vi "Upload to Sift.vi"(0 "API GRPC URL":string, 1 "Absolute Filepath":path, 5 "API Key":string, 7 "error in (no error)":errorcluster, 9 "Asset Name":string="LabVIEW-TDMS-Example", 11 "Run Name":string="TDMS Upload Example", 12 "API REST URL":string) -> (4 "Run URL":string, 15 "Error":errorcluster)   [LabVIEW 2024, in "Sift TDMS Uploader.lvlib" / "Sift TDMS Uploader.lvclass"]
doc: "Uploads TDMS file to Sift with provided Run and Asset"
uses:
  Sift TDMS Uploader.lvclass
  <vilib>/Sift/Sift/Sift API/Sift Client.lvclass
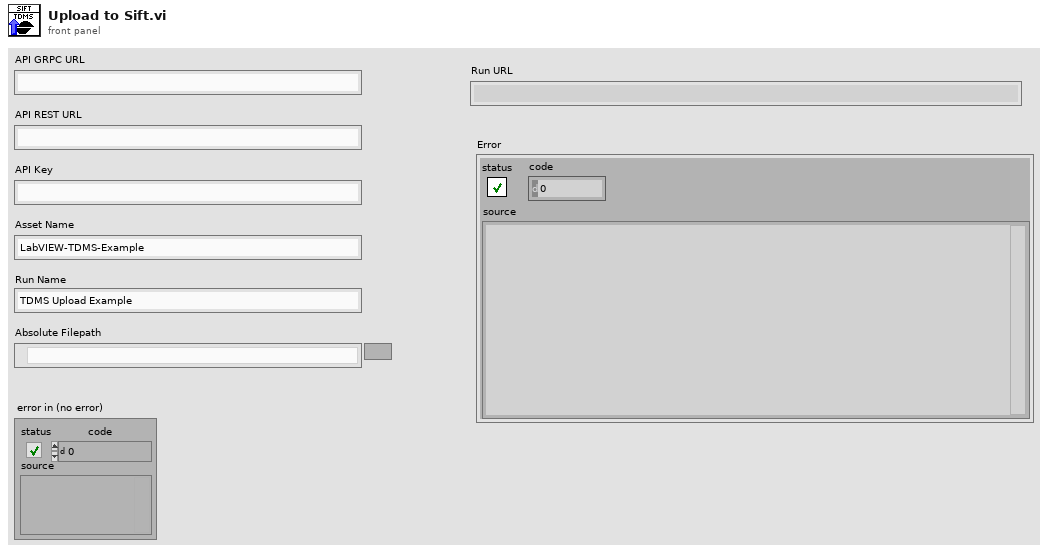
[diagram p1: front panel]
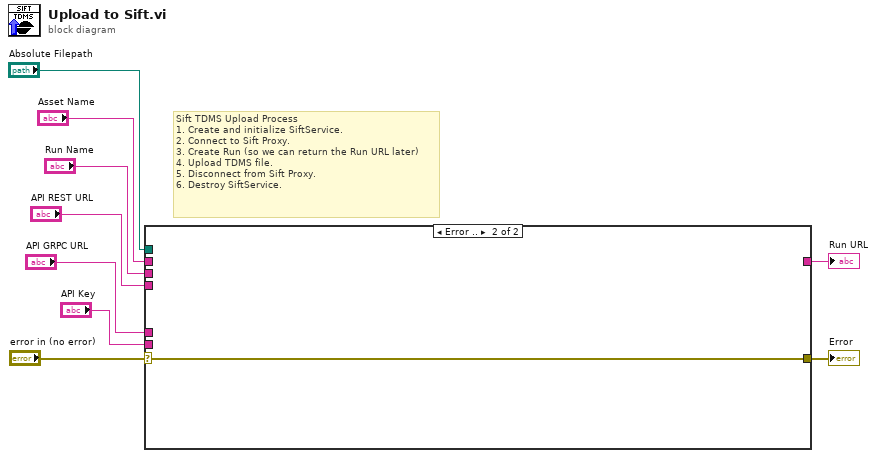
[diagram p0: block diagram]
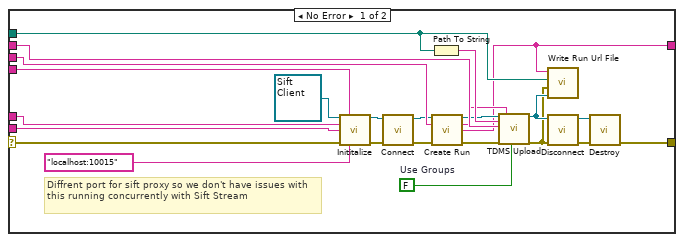
[diagram p2: hidden frame]
diagram:
  # "Sift TDMS Upload Process\n1. Create and initialize SiftService.\n2. Connect to Sift Proxy.\n3. Create Run (so we can return the Run URL later)\n4. Upload TDMS file.\n5. Disconnect from Sift Proxy.\n6. Destroy SiftService."
  n1 = case shown="Error .." "error in (no error)" {
    selector: "error in (no error)" -> [w12 w34]
    tunnel: [w32 w34] -> w9
    tunnel: "Asset Name" -> [w28 _]
    tunnel: "API GRPC URL" -> [w25 _]
    tunnel: "API Key" -> [w24 _]
    tunnel: "API REST URL" -> [w23 _]
    tunnel: "Run Name" -> [w22 _]
    tunnel: "Absolute Filepath" -> [w16 _]
    tunnel: [w15 _] -> w2
    frame No Error {
      w10 = FALSE  # Use Groups
      # "Diffrent port for sift proxy so we don't have issues with this running concurrently with Sift Stream"
      n2 = call-dynamic "Inititalize.vi"("Sift Client in"=refnum<class "Sift Client.lvclass"> refnum ("Sift Client.lvlib:Sift Client.lvclass"), "REST URL"=w23, "GRPC URL"=w25, "API Key"=w24, "error in (no error)"=w12, "Sift Proxy Address"="localhost:10015") -> ("Sift Client out"=w31:refnum<class "Sift Client.lvclass">, "error out"=w26:errorcluster)  [unwired: 8 in]
      n3 = call-dynamic "Connect.vi"("error in (no error)"=w26, "Sift Client in"=w31) -> ("error out"=w21:errorcluster, "Sift Client out"=w18:refnum<class "Sift Client.lvclass">)  [unwired: 7 in, 1 out]
      n4 = Path To String(path=w16) -> (string=w27:string)
      n5 = call-dynamic "Create Run.vi"("Sift Client in"=w18, "Name"=w22, "error in (no error)"=w21) -> ("Sift Client out"=w17:refnum<class "Sift Client.lvclass">, "Run ID"=w19:string, "URL"=w15:string, "error out"=w20:errorcluster)  [unwired: 9 in]
      n6 = call-dynamic "TDMS Upload.vi"("Sift Client in"=w17, "Filepath"=w27, "Asset Name"=w28, "error in (no error)"=w20, "Run ID"=w19, "Group Into Components"=w10) -> ("Sift Client out"=w14:refnum<class "Sift Client.lvclass">, "error out"=w13:errorcluster)  [unwired: 12 in]
      n7 = call "Write Run Url File.vi"("Sift Client in"=w14, "error in (no error)"=w13, "TDMS Filepath"=w16, "Run URL"=w15) -> ()  [unwired: 8 in]
      n8 = call-dynamic "Disconnect.vi"("error in (no error)"=w13, "Sift Client in"=w14) -> ("error out"=w29:errorcluster, "Sift Client out"=w30:refnum<class "Sift Client.lvclass">)  [unwired: 8 in]
      n9 = call-dynamic "Destroy.vi"("error in (no error)"=w29, "Sift Client in"=w30) -> ("error out"=w32:errorcluster)  [unwired: 8 in, 1 out]
    }
    frame Error {
    }
  }
  "Error" <- w9
  "Run URL" <- w2
